vi "RDS Child Receive Message.vi"(8 "error in (no error)":errorcluster, 10 "RDS Message":refnum<class "RDS Message.lvclass">, 11 "RDS State Tracker in":refnum<class "RDS State Tracker.lvclass">) -> (0 "error out":errorcluster, 3 "RDS State Tracker out":refnum<class "RDS State Tracker.lvclass">)   [LabVIEW 2015, in "RDS State Tracker.lvlib" / "RDS State Tracker.lvclass"]
uses:
  RDS State Tracker.lvclass
  Libraries/RDS Framework/RDS Message Class/RDS Message.lvclass
  Libraries/RDS Framework/RDS Message Class/RDS Message.lvclass/RDS Message.ctl
  RDS State Tracker.lvclass/RDS State Tracker.ctl
  Libraries/RDS Child Messages/AIP Status Message/AIP Status Response.lvclass
  Libraries/RDS Child Messages/AIP Status Message/AIP Status Response.lvclass/AIP Status Response.ctl
  RDS State/RDS State.lvclass/RDS State.ctl
  Libraries/RDS Child Messages/GPS Data Message/GPS Data Message.lvclass
  Libraries/RDS Child Messages/GPS Data Message/GPS Data Message.lvclass/GPS Data Message.ctl
  Libraries/RDS Child Messages/MCB/MCB Status Message/MCB Status.lvclass
  Libraries/RDS Child Messages/MCB/MCB Status Message/MCB Status.lvclass/MCB Status.ctl
  Libraries/RDS Child Messages/Compass/Compass Data Message.lvclass
  Libraries/RDS Child Messages/Compass/Compass Data Message.lvclass/Compass Data Message.ctl
  Libraries/RDS Child Messages/Depth Data Message/Depth Data Message.lvclass
  Libraries/RDS Child Messages/Depth Data Message/Depth Data Message.lvclass/Depth Data Message.ctl
  Libraries/RDS Child Messages/Battery Data/Battery Message.lvclass
  Libraries/RDS Child Messages/Battery Data/Battery Message.lvclass/Battery Message.ctl
  Libraries/RDS Child Messages/Mission Messages/Mission Controller State Message.lvclass
  Libraries/RDS Child Messages/Mission Messages/Mission Controller State Message.lvclass/Mission Controller State Message.ctl
  Libraries/RDS Child Messages/Helm/Helm Status Message/Helm Status Message.lvclass
  Libraries/RDS Child Messages/Helm/Helm Status Message/Helm Status Message.lvclass/Helm Status Message.ctl
  Libraries/RDS Child Messages/Controller State Message/Controller State.lvclass
  Libraries/RDS Child Messages/Controller State Message/Controller State.lvclass/Controller State.ctl
  Libraries/RDS Child Messages/State Sample Message/State Sample Message.lvclass
  Libraries/RDS Framework/RDS Message ID.ctl
  Libraries/RDS Child Messages/State Sample Message/State Sample Message.lvclass/State Sample Message.ctl
  Libraries/RDS Serial Handler/RDS Serial Frame.lvclass
  RDS State/RDS State.lvclass
  Actors/RDS Parent Actor/RDS Parent Actor/RDS Parent Actor.lvclass
  Libraries/RDS Child Messages/RDS Child Messages.lvlib
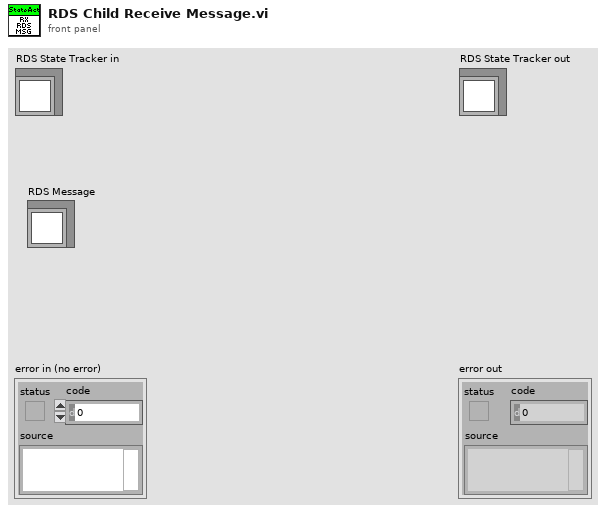
[diagram p1: front panel]
types:
  T1 = typedef "RDS Child Messages.lvlib/RDS Message ID.ctl" = enum16{"RDS Hello World", "String Message", "AIP_Status", "AIP_Command", "GPS_Data", "MCB_Command", "MCB_Status", "Compass_Data", "Depth_Data", "Battery_Data", "Contoller_State", "Set_Mag_Dev", "BTB_Shutdown", "State_Sample_Request", "State_Sample", "PID_Gains_Set", "Helm_Limiter_Set", "Helm_Heading_Command", "Helm_Steering_Command", "Helm_Status", "Controller_Message", "AIP_Set_Min_Depth", "Mission_Controller_State", "Mission_Upload", "Mission_Set_Op_and_Run", "Mission_Settings_Set"}
  T2 = typedef "RDS Instrument Library.lvlib/AIP Status.ctl" = cluster{"FWD Port":T3, "FWD Stbd":T3, "AFT Port":T3, "AFT Stbd":T3, "AIP Depth Min":u8}
  T3 = typedef "RDS Instrument Library.lvlib/AIP States.ctl" = enum16{"Deploy", "Deploying", "Deployed", "Stow", "Stowing", "Stowed", "Fault", "brakeOnStow", "breakOnDeploy", "Stopped", "Stopping"}
  T4 = typedef "RDS Libraries.lvlib/NMEA.lvlib/NMEA_GPRMC-data.ctl" = cluster{"TimeStamp":timestamp, "Validity":bool, "Latitude":dbl, "Latitude-Direction":T5, "Longitude":dbl, "Longitude-Direction":T6, "Speed in knots":sgl, "True course":sgl, "Date Stamp":timestamp, "Magnetic Variation (East/West)":sgl, "GPS Latitude":dbl, "GPS Longitude":dbl}
  T5 = typedef "RDS Libraries.lvlib/NMEA.lvlib/NMEA_LatitudeDirection.ctl" = enum16{"", "North", "South"}
  T6 = typedef "RDS Libraries.lvlib/NMEA.lvlib/NMEA_LongitudeDirection.ctl" = enum16{"", "East", "West"}
  T7 = typedef "RDS Child Messages.lvlib/MCB Motor Status.ctl" = cluster{"Motor Power":i16, "Motor Command":i16, "Battery Volts":sgl, "Battery Amps":sgl, "Motor Amps":sgl, "MCU Temp":i16, "Heatsink Temp":i16, "Fault Flags":u16, "StatusFlags":u16}
  T8 = typedef "RDS Child Messages.lvlib/MCB Channel.ctl" = enum16{"PORT", "STBD"}
  T9 = typedef "RDS Instrument Library.lvlib/Compass Data.ctl" = cluster{"Compass Heading":sgl, "pitch Angle":sgl, "roll Angle":sgl, "Temperature":sgl, "Depth":sgl, "Magnetic Field":sgl, "Magnetic Field X":sgl, "Magnetic Field Y":sgl, "Magnetic Field Z":sgl, "Acceleration":sgl, "Acceleration X":sgl, "Acceleration Y":sgl, "Gyro":sgl, "Gyro X":sgl, "Acceleration Z":sgl, "Gyro Y":sgl, "Raw Heading":sgl}
  T10 = typedef "RDS Child Messages.lvlib/Depth Data.ctl" = cluster{"Depth":sgl, "Water Temp":i8}
  T11 = typedef "RDS Instrument Library.lvlib/Battery Data.ctl" = cluster{"Battery Status":T12, "Pack Voltage":sgl, "Pack Current":sgl, "Pack Capacity":sgl, "Max Cell Temp":sgl, "Min Cell Temp":sgl, "Max Cell Voltage":sgl, "Min Cell Voltage":sgl}
  T12 = typedef "RDS Instrument Library.lvlib/Battery Status.ctl" = enum16{"Pack Normal", "Alarm: Cell temp too high", "Alarm: Pack voltage too high", "Warn: Pack voltage too high ", "Alarm: Pack voltage too low", "Warn: Pack voltage low", "Alarm Pack current too high", "Warn: Pack current too high ", "Fault: Pack to chassis connection detected", "Fault: Pack to cell connection error", "Fautl: System error"}
  T13 = typedef "RDS Child Messages.lvlib/Mission Controller State Message.lvclass/Mission Controller State Control.ctl" = cluster{"iHasControl":bool, "controlTimer":timestamp, "Nav State":T14, "Current MissionOp Index":i32, "Mission":T15[], "Distance to Target":dbl, "Seconds to Timeout":dbl}
  T14 = typedef "RDS Mission Controller Actor.lvlib/Mission Controller Navigation State.ctl" = cluster{"GPS Latitude":ext, "GPS Longitude":ext, "Compass Heading":dbl, "Speed":dbl}
  T15 = typedef "RDS Mission Controller Actor.lvlib/MissionOp.ctl" = cluster{"MissionOp Type":enum16{"Waypoint", "Loiter", "Wait", "Deploy AIP", "Stow AIP"}, "Duration (s)":u16, "Throttle":i16, "GPS Latitude":dbl, "GPS Longitude":dbl, "Loiter Range (m)":u16}
  T16 = typedef "RDS Child Messages.lvlib/Helm Status Control.ctl" = cluster{"Helm State":T17, "Heading Command Control":T18, "Steering Command Control":T19, "Last Command Time":timestamp, "Gains":T20, "Current Heading":dbl, "Port Throttle":i16, "STBD Throttle":i16, "Limiter":dbl}
  T17 = typedef "RDS Helm Actor.lvlib/Helm State.ctl" = enum16{"Idle", "Executing Heading Command", "Executing Steering Command"}
  T18 = typedef "RDS Child Messages.lvlib/Heading Command Cntrl.ctl" = cluster{"Throttle":i16, "Heading":sgl, "Duration (s)":i16}
  T19 = typedef "RDS Child Messages.lvlib/Steering Command Cntrl.ctl" = cluster{"Throttle":i16, "Rudder":i8, "Duration (s)":u16}
  T20 = typedef "RDS Child Messages.lvlib/PID Gains Control.ctl" = cluster{"P (Kc)":sgl, "I (Ti)":sgl, "D (Td)":sgl}
  T21 = typedef "RDS Controller Actor.lvlib/Controller.ctl" = enum16{"Idle", "Local Remote Control", "Shore Remote Control", "Mission Control"}
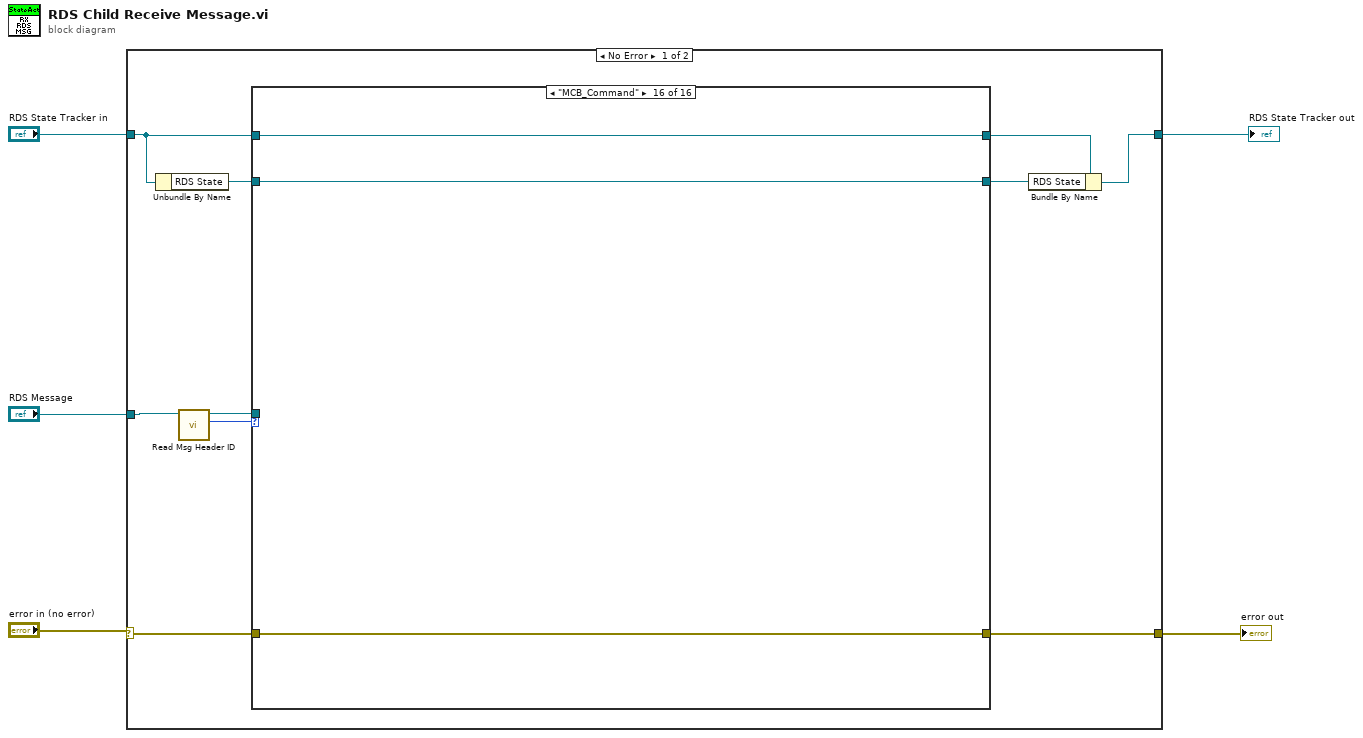
[diagram p0: block diagram]
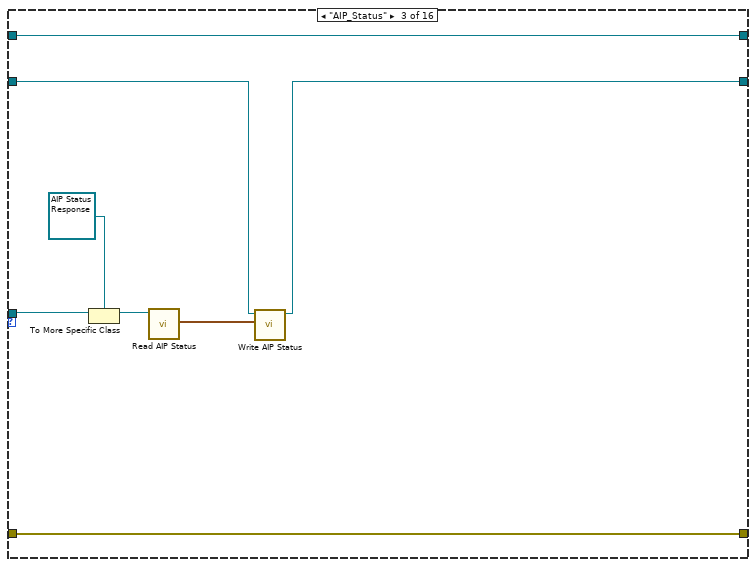
[diagram p4: hidden frame]
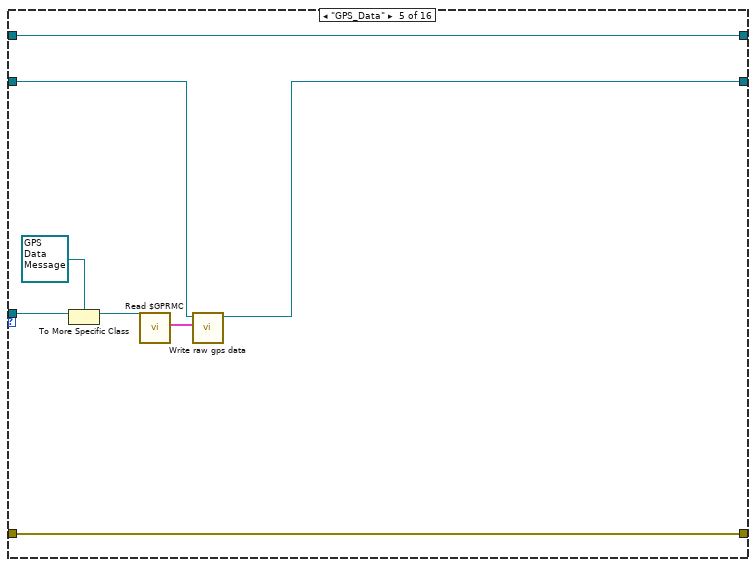
[diagram p6: hidden frame]
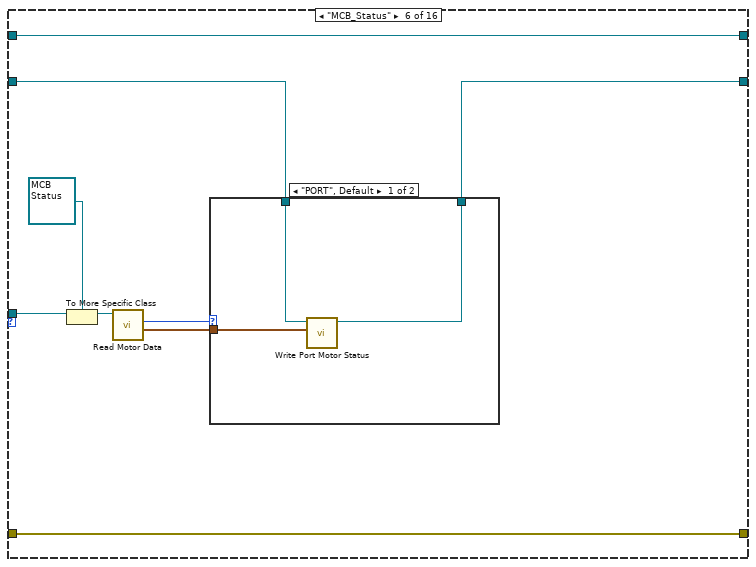
[diagram p7: hidden frame]
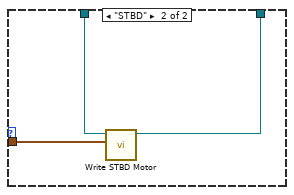
[diagram p8: hidden frame]
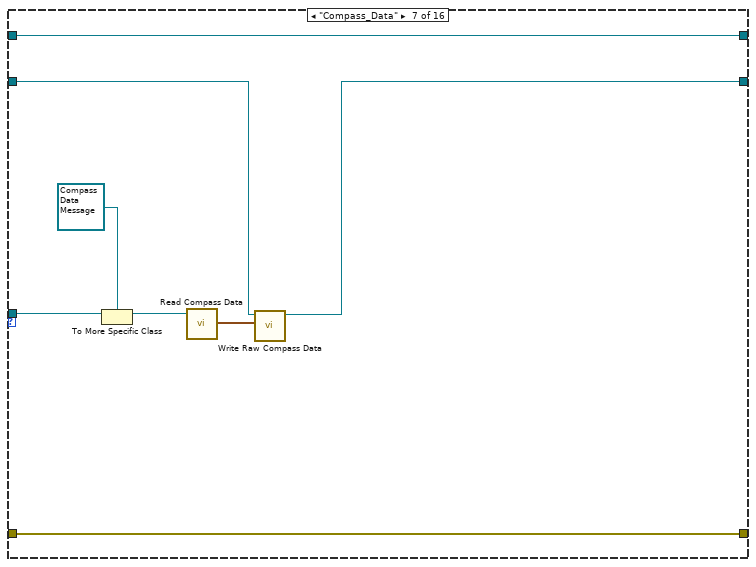
[diagram p9: hidden frame]
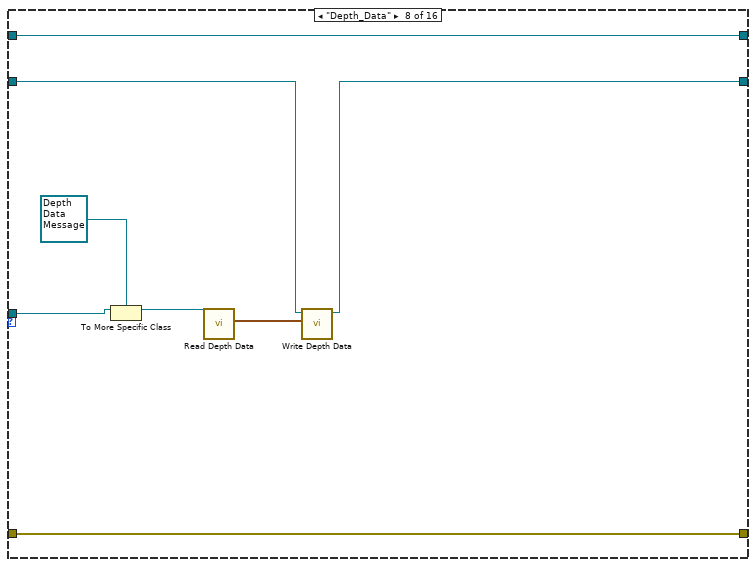
[diagram p10: hidden frame]
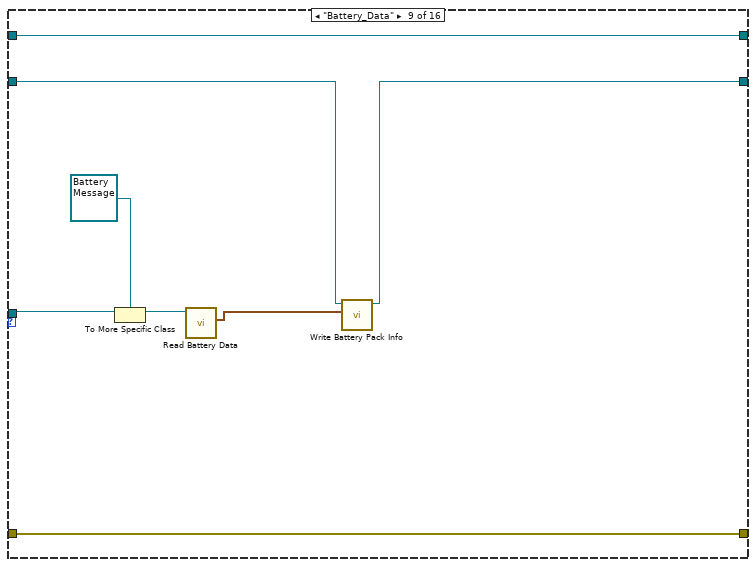
[diagram p11: hidden frame]
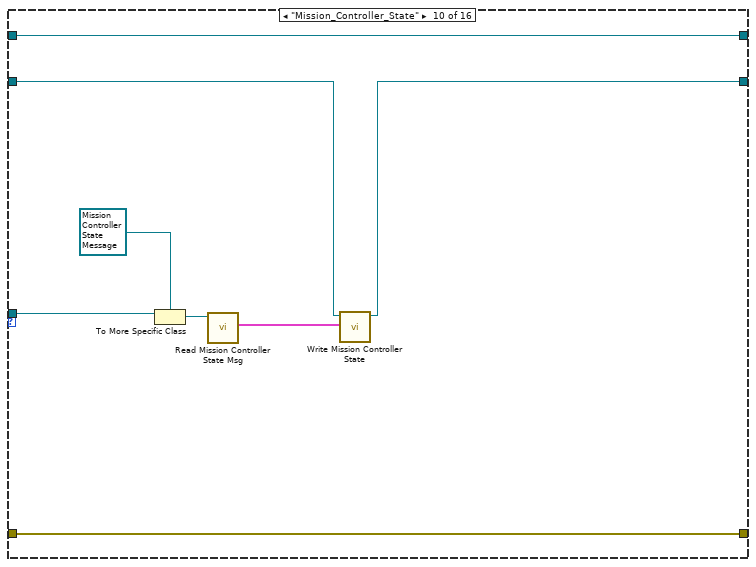
[diagram p12: hidden frame]
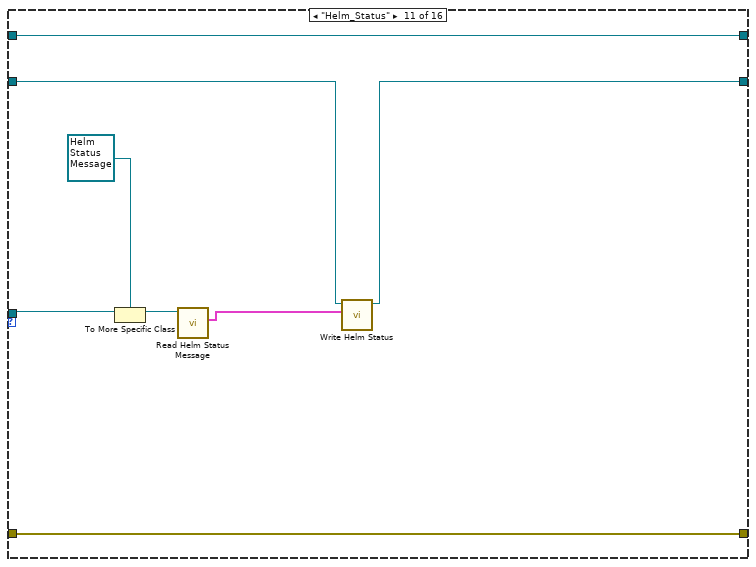
[diagram p13: hidden frame]
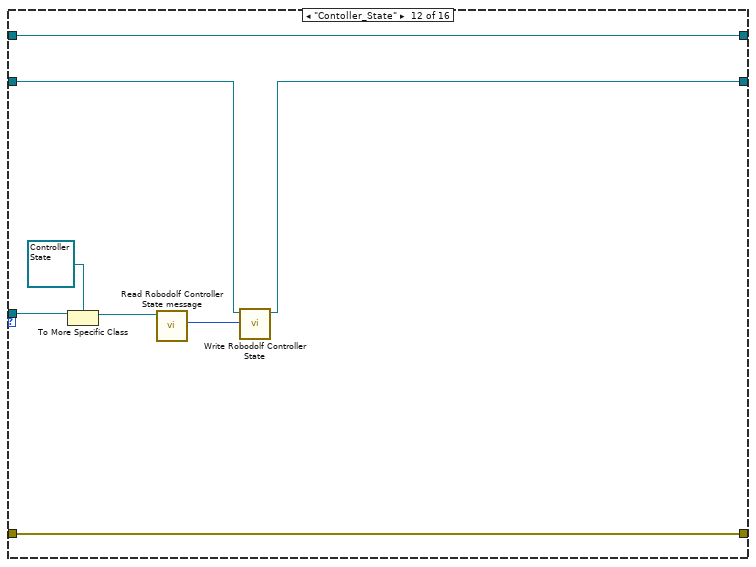
[diagram p14: hidden frame]
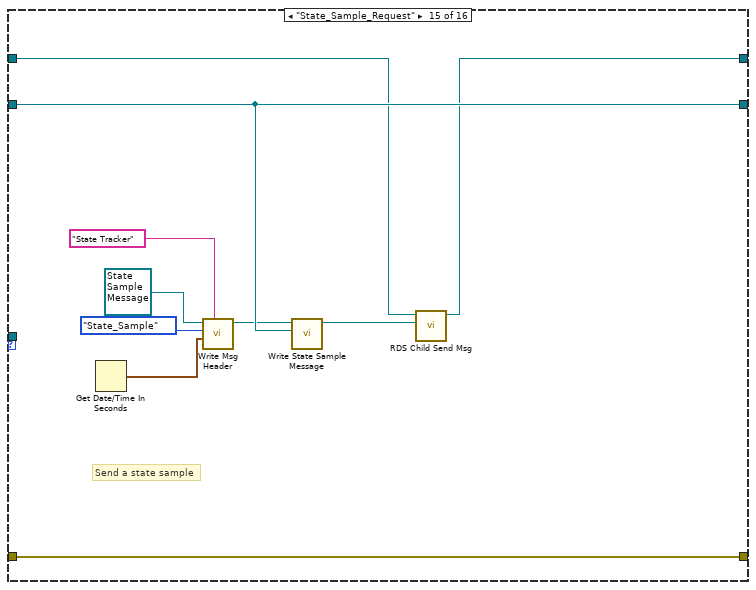
[diagram p17: hidden frame]
diagram:
  n1 = case shown="No Error" "error in (no error)" {
    selector: "error in (no error)" -> [w8 w123]
    tunnel: "RDS Message" -> [w15 _]
    tunnel: "RDS State Tracker in" -> [w7 w124]
    tunnel: [w10 w124] -> w2
    tunnel: [w9 w123] -> w1
    frame No Error {
      n2 = Unbundle By Name(w7) -> ("RDS State"=w12:refnum<class "RDS State.lvclass">)
      n3 = call "Read Msg Header ID.vi"("RDS Message in"=w15) -> ("Msg ID"=w14:T1, "RDS Message out"=w13:refnum<class "RDS Message.lvclass">)  [unwired: 6 in, 3 out]
      n4 = case shown="\"MCB_Command\"" w14 {
        tunnel: w13 -> [_ _ w29 _ w40 w49 w62 w69 w78 w85 w95 w103 _ _ _ _]
        tunnel: w12 -> [w18 w21 w25 w32 w37 w44 w59 w68 w75 w82 w90 w99 w105 w108 w118 w121]
        tunnel: [w18 w21 w24 w32 w33 w43 w56 w66 w74 w81 w89 w98 w105 w108 w118 w121] -> w11
        tunnel: [w17 w20 w23 w31 w36 w42 w58 w65 w73 w87 w94 w97 w106 w109 w119 w122] -> w9
        tunnel: w8 -> [w17 w20 w23 w31 w36 w42 w58 w65 w73 w87 w94 w97 w106 w109 w119 w122]
        tunnel: w7 -> [w16 w19 w22 w30 w34 w41 w57 w64 w72 w86 w93 w96 w104 w107 w111 w120]
        tunnel: [w16 w19 w22 w30 w34 w41 w57 w64 w72 w86 w93 w96 w104 w107 w110 w120] -> w6
        frame "RDS Hello World", Default {
        }
        frame "String Message" {
        }
        frame "AIP_Status" {
          n5 = To More Specific Class(target class=refnum<class "AIP Status Response.lvclass"> refnum ("RDS Child Messages.lvlib:AIP Status Response.lvclass"), reference=w29) -> (specific class reference=w27:refnum<class "AIP Status Response.lvclass">)  [unwired: 1 in, 1 out]
          n6 = call "Read AIP Status.vi"("AIP Status Response in"=w27) -> ("AIP Status"=w26:T2)  [unwired: 7 in, 3 out]
          n7 = call "Write AIP Status.vi"("AIP Status"=w26, "RDS State in"=w25) -> ("RDS State out"=w24:refnum<class "RDS State.lvclass">)  [unwired: 8 in, 1 out]
        }
        frame "AIP_Command" {
          # "I'm not recording this."
        }
        frame "GPS_Data" {
          n8 = To More Specific Class(target class=refnum<class "GPS Data Message.lvclass"> refnum ("RDS Child Messages.lvlib:GPS Data Message.lvclass"), reference=w40) -> (specific class reference=w38:refnum<class "GPS Data Message.lvclass">)  [unwired: 1 in, 1 out]
          n9 = call "Read $GPRMC.vi"("GPS Data Message in"=w38) -> ("GPRMC-data"=w35:T4)  [unwired: 8 in, 2 out]
          n10 = call "Write raw gps data.vi"("GPRMC-data"=w35, "RDS State in"=w37) -> ("RDS State out"=w33:refnum<class "RDS State.lvclass">)  [unwired: 8 in, 1 out]
        }
        frame "MCB_Status" {
          n11 = To More Specific Class(target class=refnum<class "MCB Status.lvclass"> refnum ("RDS Child Messages.lvlib:MCB Status.lvclass"), reference=w49) -> (specific class reference=w47:refnum<class "MCB Status.lvclass">)  [unwired: 1 in, 1 out]
          n12 = call "Read Motor Data.vi"("MCB Status in"=w47) -> ("Motor Data"=w45:T7, "Motor"=w46:T8)  [unwired: 7 in, 2 out]
          n13 = case shown="\"PORT\", Default" w46 {
            tunnel: w45 -> [w51 w55]
            tunnel: w44 -> [w52 w54]
            tunnel: [w50 w53] -> w43
            frame "PORT", Default {
              n14 = call "Write Port Motor Status.vi"("Port Motor Status"=w51, "RDS State in"=w52) -> ("RDS State out"=w50:refnum<class "RDS State.lvclass">)  [unwired: 8 in, 1 out]
            }
            frame "STBD" {
              n15 = call "Write STBD Motor.vi"("STBD Motor"=w55, "RDS State in"=w54) -> ("RDS State out"=w53:refnum<class "RDS State.lvclass">)  [unwired: 8 in, 1 out]
            }
          }
        }
        frame "Compass_Data" {
          n16 = To More Specific Class(target class=refnum<class "Compass Data Message.lvclass"> refnum ("RDS Child Messages.lvlib:Compass Data Message.lvclass"), reference=w62) -> (specific class reference=w61:refnum<class "Compass Data Message.lvclass">)  [unwired: 1 in, 1 out]
          n17 = call "Read Compass Data.vi"("Compass Data Message in"=w61) -> ("Compass Data"=w60:T9)  [unwired: 8 in, 2 out]
          n18 = call "Write Raw Compass Data.vi"("Compass Data"=w60, "RDS State in"=w59) -> ("RDS State out"=w56:refnum<class "RDS State.lvclass">)  [unwired: 8 in, 1 out]
        }
        frame "Depth_Data" {
          n19 = To More Specific Class(target class=refnum<class "Depth Data Message.lvclass"> refnum ("RDS Child Messages.lvlib:Depth Data Message.lvclass"), reference=w69) -> (specific class reference=w70:refnum<class "Depth Data Message.lvclass">)  [unwired: 1 in, 1 out]
          n20 = call "Read Depth Data.vi"("Depth Data Message in"=w70) -> ("Depth Data"=w67:T10)  [unwired: 8 in, 2 out]
          n21 = call "Write Depth Data.vi"("Depth Data"=w67, "RDS State in"=w68) -> ("RDS State out"=w66:refnum<class "RDS State.lvclass">)  [unwired: 8 in, 1 out]
        }
        frame "Battery_Data" {
          n22 = To More Specific Class(target class=refnum<class "Battery Message.lvclass"> refnum ("RDS Child Messages.lvlib:Battery Message.lvclass"), reference=w78) -> (specific class reference=w77:refnum<class "Battery Message.lvclass">)  [unwired: 1 in, 1 out]
          n23 = call "Read Battery Data.vi"("Battery Message in"=w77) -> ("Battery Pack Info"=w76:T11)  [unwired: 8 in, 2 out]
          n24 = call "Write Battery Pack Info.vi"("Battery Pack Info"=w76, "RDS State in"=w75) -> ("RDS State out"=w74:refnum<class "RDS State.lvclass">)  [unwired: 8 in, 1 out]
        }
        frame "Mission_Controller_State" {
          n25 = To More Specific Class(target class=refnum<class "Mission Controller State Message.lvclass"> refnum ("RDS Child Messages.lvlib:Mission Controller State Message.lvclass"), reference=w85) -> (specific class reference=w83:refnum<class "Mission Controller State Message.lvclass">)  [unwired: 1 in, 1 out]
          n26 = call "Read Mission Controller State Msg.vi"("Mission Controller State Message in"=w83) -> ("Mission Controller State"=w80:T13)  [unwired: 8 in, 2 out]
          n27 = call "Write Mission Controller State.vi"("Mission Controller State"=w80, "RDS State in"=w82) -> ("RDS State out"=w81:refnum<class "RDS State.lvclass">)  [unwired: 8 in, 1 out]
        }
        frame "Helm_Status" {
          n28 = To More Specific Class(target class=refnum<class "Helm Status Message.lvclass"> refnum ("RDS Child Messages.lvlib:Helm Status Message.lvclass"), reference=w95) -> (specific class reference=w91:refnum<class "Helm Status Message.lvclass">)  [unwired: 1 in, 1 out]
          n29 = call "Read Helm Status Message.vi"("Helm Status Message in"=w91) -> ("Helm Status"=w88:T16)  [unwired: 8 in, 2 out]
          n30 = call "Write Helm Status.vi"("Helm Status"=w88, "RDS State in"=w90) -> ("RDS State out"=w89:refnum<class "RDS State.lvclass">)  [unwired: 8 in, 1 out]
        }
        frame "Contoller_State" {
          n31 = To More Specific Class(target class=refnum<class "Controller State.lvclass"> refnum ("RDS Child Messages.lvlib:Controller State.lvclass"), reference=w103) -> (specific class reference=w101:refnum<class "Controller State.lvclass">)  [unwired: 1 in, 1 out]
          n32 = call "Read Robodolf Controller State message.vi"("Controller State in"=w101) -> ("Controller State"=w100:T21)  [unwired: 8 in, 2 out]
          n33 = call "Write Robodolf Controller State.vi"("Controller State"=w100, "RDS State in"=w99) -> ("RDS State out"=w98:refnum<class "RDS State.lvclass">)  [unwired: 8 in, 1 out]
        }
        frame "Set_Mag_Dev" {
        }
        frame "BTB_Shutdown" {
        }
        frame "State_Sample_Request" {
          # "Send a state sample"
          n34 = Get Date/Time In Seconds() -> (seconds since 1Jan1904=w114:timestamp)
          n35 = call "Write Msg Header.vi"("Sender Name"="State Tracker", "Time Stamp"=w114, "Msg ID"=RDS_Message_ID."State_Sample", "RDS Message in"=refnum<class "State Sample Message.lvclass"> refnum ("RDS Child Messages.lvlib:State Sample Message.lvclass")) -> ("RDS Message out"=w113:refnum<class "State Sample Message.lvclass">)  [unwired: 6 in, 1 out]
          n36 = call "Write State Sample Message.vi"("RDS State Tracker.lvlib:RDS State.lvclass"=w118, "State Sample Message in"=w113) -> ("State Sample Message out"=w112:refnum<class "State Sample Message.lvclass">)  [unwired: 8 in, 1 out]
          n37 = call "RDS Child Send Msg.vi"("RDS Message"=w112, "RDS Parent Actor in"=w111) -> ("RDS Parent Actor out"=w110:refnum<class "RDS State Tracker.lvclass">)  [unwired: 8 in, 1 out]
        }
        frame "MCB_Command" {
        }
      }
      n38 = Bundle By Name(cluster=w6, "RDS State"=w11) -> (w10:refnum<class "RDS State Tracker.lvclass">)
    }
    frame Error {
    }
  }
  "error out" <- w1
  "RDS State Tracker out" <- w2
